vi "Set Family.vi"(8 "error in (no error)":errorcluster, 10 "family":T1, 11 "DOM document in":refnum<k20>) -> (0 "error out":errorcluster, 3 "DOM document out":refnum<k20>)   [LabVIEW 2017, in "Error File Management.lvlib"]
uses:
  Error File Management.lvlib
  Controls/NI Family.ctl
  <vilib>/xml/Close Reference(Node).vi
  <vilib>/xml/NI_XML.lvlib
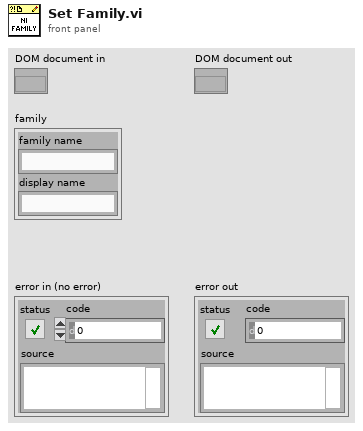
[diagram p1: front panel]
types:
  T1 = typedef "Error File Management.lvlib/NI Family.ctl" = cluster{"family name":string, "display name":string}
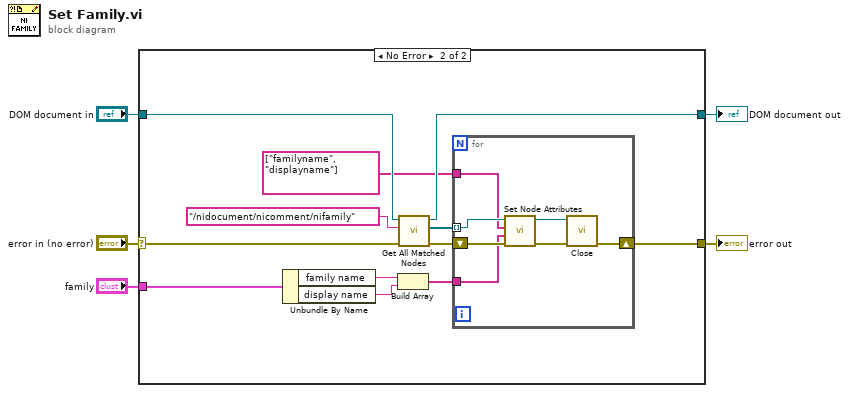
[diagram p0: block diagram]
diagram:
  n1 = case shown="No Error" "error in (no error)" {
    selector: "error in (no error)" -> [w7 w13]
    tunnel: [w6 w19] -> w5
    tunnel: "DOM document in" -> [w6 w18]
    tunnel: [w7 w14] -> w2
    tunnel: "family" -> [_ w10]
    frame Error {
    }
    frame No Error {
      n2 = Unbundle By Name(w10) -> ("family name"=w9:string, "display name"=w8:string)
      n3 = Build Array(w9, w8) -> (w12:string[])
      n4 = call <vilib>:"Get All Matched Nodes.vi"("error in (no error)"=w13, "XPath expression"="/nidocument/nicomment/nifamily", "node in"=w18) -> ("error out"=w17:errorcluster, "node result array"=w16:refnum<k20>[], "node out"=w19:refnum<k20>)  [unwired: 6 in]
      n5 = for {
        tunnel: w16 -> [w24] mode=indexing
        shift-right: [w25] -> w14
        shift-left: w17 -> [w26]
        tunnel: w12 -> [w23]
        tunnel: string[] ["familyname", "displayname"] ("names") -> [w20]
        n6 = call "Set Node Attributes.vi"("error in (no error)"=w26, "values"=w23, "names"=w20, "node in"=w24) -> ("error out"=w21:errorcluster, "node out"=w22:refnum<k20>)  [unwired: 6 in]
        n7 = call-poly <vilib>:"Close.vi"("error in (no error)"=w21, "node"=w22) -> ("error out"=w25:errorcluster)  [unwired: 7 out]
      }
    }
  }
  "DOM document out" <- w5
  "error out" <- w2
